vi "Change all terminals to Required.vi"(8 "error in":errorcluster, 11 "VI ref to change":refnum<vi>) -> (0 "error out":errorcluster, 3 "VI ref (dup)":refnum<vi>)   [LabVIEW 2013]
panel:
  out "Controls":string[](array[string])
  out "WiringRules[] after":T1(array[ring])
  out "Control?\n (otherwise indicator, \nor not hooked up)":enum8{"False", "True", "Mixed"}[](array[numeric])
  out "WiringRules[] before":T1(array[ring])
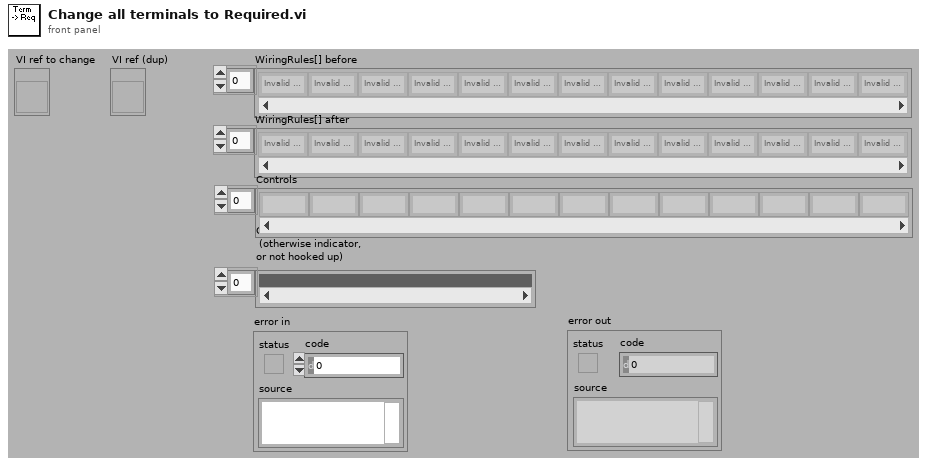
[diagram p1: front panel]
types:
  T1 = enum16{"Invalid Wire Rule", "Required", "Recommended", "Optional", "Dynamic Dispatch"}[]
  T2 = enum16{"Invalid Wire Rule", "Required", "Recommended", "Optional", "Dynamic Dispatch"}
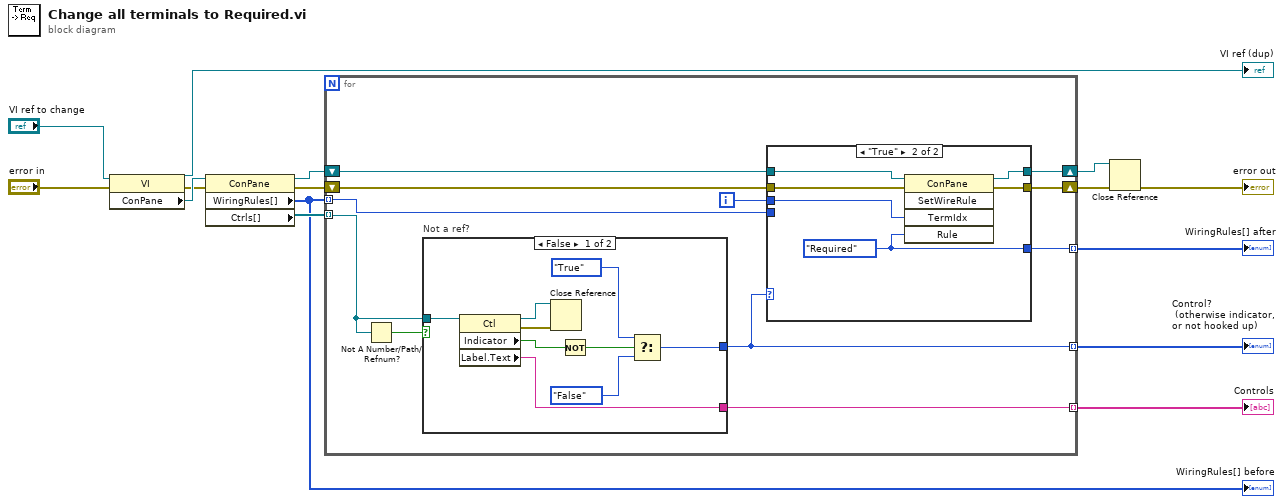
[diagram p0: block diagram]
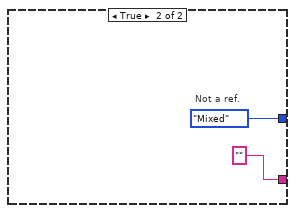
[diagram p2: hidden frame]
diagram:
  n1 = property class="VI"(reference="VI ref to change", error in="error in") -> (reference out=→"VI ref (dup)":refnum<vi>, error out=w12:errorcluster, "ConPane"=w15:refnum<vi>)
  n2 = property class="ConPane"(reference=w15, error in=w12) -> (reference out=w3:refnum<vi>, error out=w4:errorcluster, "WiringRules[]"=w5:T1, "Ctrls[]"=w13:refnum<vi>[])
  "WiringRules[] before" <- w5
  n3 = for {
    tunnel: w13 -> [w23] mode=indexing
    tunnel: [w26] -> w14 mode=indexing
    tunnel: w5 -> [w25] mode=indexing
    tunnel: [w24] -> w10 mode=indexing
    tunnel: [w21] -> w6 mode=indexing
    shift-right: [w19] -> w1
    shift-left: w4 -> [w18]
    shift-right: [w16] -> w2
    shift-left: w3 -> [w17]
    i -> [w20]
    n4 = Not A Number/Path/Refnum?(number/path/refnum=w23) -> (NaN/Path/Refnum?=w22:bool)
    n5 = case "Not a ref?" shown="False" w22 {
      tunnel: [w34 enum8{"False", "True", "Mixed"}."Mixed" ("Indicator")] -> w26
      tunnel: w23 -> [w31 _]
      tunnel: [w27 "" ("Label.Text")] -> w21
      frame False {
        n6 = property class="Ctl"(reference=w31) -> (reference out=w32:refnum<vi>, error out=w30:errorcluster, "Indicator"=w35:bool, "Label.Text"=w27:string)  [unwired: 1 in]
        n7 = Close Reference(reference=w32, error in (no error)=w30) -> ()  [unwired: 1 out]
        n8 = Not(x=w35) -> (.not. x?=w33:bool)
        n9 = Select(t=enum8{"False", "True", "Mixed"}."True" ("Indicator"), s=w33, f=enum8{"False", "True", "Mixed"}."False" ("Indicator")) -> (s? t:f=w34:enum8{"False", "True", "Mixed"})
      }
      frame True {
        # "Not a ref."
      }
    }
    n10 = case shown="\"True\"" w26 {
      tunnel: w25 -> [w40 _]
      tunnel: [w40 w45] -> w24
      tunnel: w20 -> [_ w46]
      tunnel: [w38 w44] -> w19
      tunnel: w18 -> [w38 w43]
      tunnel: w17 -> [w39 w42]
      tunnel: [w39 w41] -> w16
      frame "False", "Mixed" {
      }
      frame "True" {
        w45 = T2."Required" ("Wire Rule")
        n11 = invoke class="ConPane" method="SetWireRule"(reference=w42, error in=w43, "TermIdx"=w46, "Rule"=w45) -> (reference out=w41:refnum<vi>, error out=w44:errorcluster)  [unwired: 1 in, 3 out]
      }
    }
  }
  "Control?\n (otherwise indicator, \nor not hooked up)" <- w14
  "WiringRules[] after" <- w10
  "Controls" <- w6
  n12 = Close Reference(reference=w2, error in (no error)=w1) -> (error out=→"error out":errorcluster)
